vi "add2Parameter.vi"(0 "Enum":T1(ring), 1 "data":variant, 2 "Parameter":variant, 3 "typeDescriptor":string, 5 "error in":errorcluster) -> (16 "Parameter out":variant, 17 "typeDescriptor out":string, 19 "error out":errorcluster)   [LabVIEW 2012, in "HGF_SV.lvlib"]
uses:
  HGF_SV.lvlib
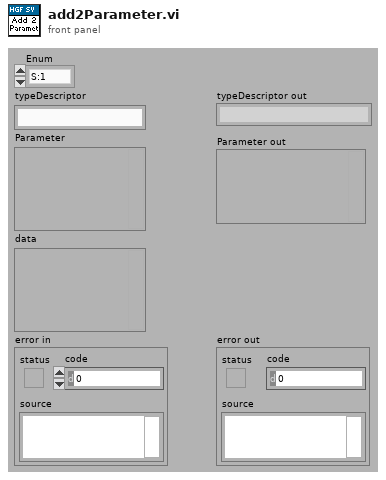
[diagram p1: front panel]
types:
  T1 = enum16{"S:1", "S:2", "L:1", "L:2", "I:1", "I:2", "X:1", "X:2", "F:1", "F:2", "D:1", "D:2", "C"}
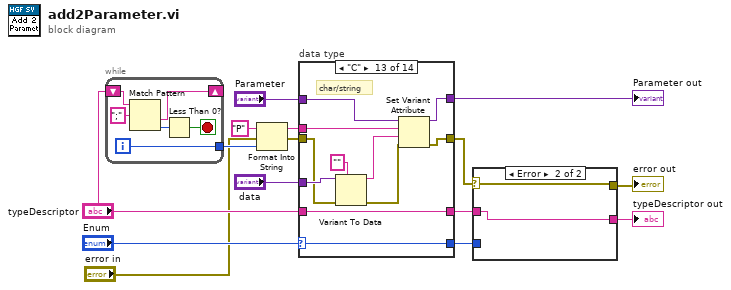
[diagram p0: block diagram]
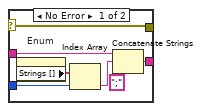
[diagram p2: hidden frame]
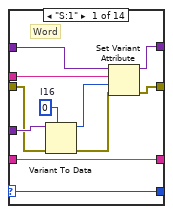
[diagram p3: hidden frame]
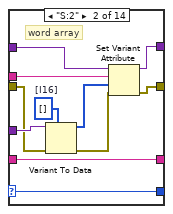
[diagram p4: hidden frame]
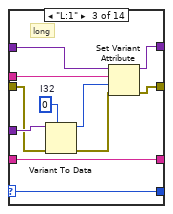
[diagram p5: hidden frame]
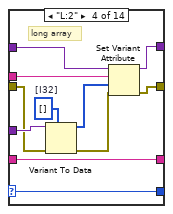
[diagram p6: hidden frame]
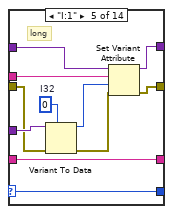
[diagram p7: hidden frame]
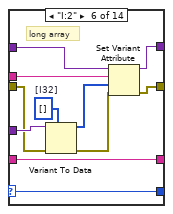
[diagram p8: hidden frame]
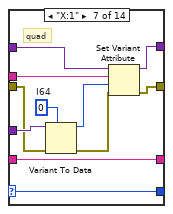
[diagram p9: hidden frame]
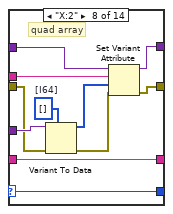
[diagram p10: hidden frame]
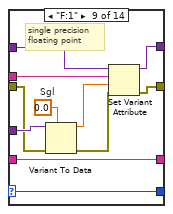
[diagram p11: hidden frame]
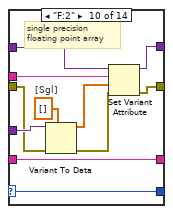
[diagram p12: hidden frame]
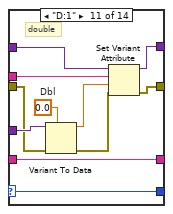
[diagram p13: hidden frame]
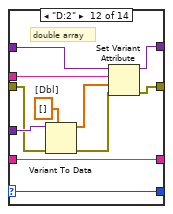
[diagram p14: hidden frame]
diagram:
  n1 = while {
    shift-right: [w19] -> _
    shift-left: "typeDescriptor" -> [w21]
    tunnel: [w16] -> w12
    i -> [w16]
    stop <- w17 stop-if-true
    n2 = Match Pattern(string=w21, regular expression=";") -> (after substring=w19:string, offset past match=w18:i32)  [unwired: 3 out]
    n3 = Less Than 0?(x=w18) -> (x < 0?=w17:bool)
  }
  n4 = Format Into String(initial string="P", error in="error in", w12) -> (resulting string=w10:string, error out=w9:errorcluster)  [unwired: 1 in]
  n5 = case "data type" shown="\"C\"" "Enum" {
    selector: "Enum" -> [w23 w33 w45 w55 w67 w77 w89 w99 w111 w121 w133 w143 w155 w166]
    tunnel: "data" -> [w30 w41 w52 w63 w74 w85 w96 w107 w118 w129 w140 w151 w162 _]
    tunnel: "Parameter" -> [w32 w43 w54 w65 w76 w87 w98 w109 w120 w131 w142 w153 w164 w168]
    tunnel: w10 -> [w31 w42 w53 w64 w75 w86 w97 w108 w119 w130 w141 w152 w163 _]
    tunnel: w9 -> [w28 w38 w50 w60 w72 w82 w94 w104 w116 w126 w138 w148 w160 w165]
    tunnel: [w26 w36 w48 w58 w70 w80 w92 w102 w114 w124 w136 w146 w158 w168] -> w5
    tunnel: [w25 w35 w47 w57 w69 w79 w91 w101 w113 w123 w135 w145 w157 w165] -> w4
    tunnel: "typeDescriptor" -> [w24 w34 w46 w56 w68 w78 w90 w100 w112 w122 w134 w144 w156 w167]
    tunnel: [w24 w34 w46 w56 w68 w78 w90 w100 w112 w122 w134 w144 w156 w167] -> w6
    tunnel: [w23 w33 w45 w55 w67 w77 w89 w99 w111 w121 w133 w143 w155 w166] -> w7
    frame "S:1" {
      w22 = i16 0  # I16
      # "Word"
      n6 = Variant To Data(error in=w28, type=w22, Variant=w30) -> (data=w29:i16, error out=w27:errorcluster)
      n7 = Set Variant Attribute(Variant=w32, name=w31, value=w29, error in=w27) -> (Variant out=w26:variant, error out=w25:errorcluster)  [unwired: 1 out]
    }
    frame "S:2" {
      w40 = i16[] []  # [I16]
      # "word array"
      n8 = Variant To Data(error in=w38, type=w40, Variant=w41) -> (data=w39:i16[], error out=w37:errorcluster)
      n9 = Set Variant Attribute(Variant=w43, name=w42, value=w39, error in=w37) -> (Variant out=w36:variant, error out=w35:errorcluster)  [unwired: 1 out]
    }
    frame "L:1" {
      w44 = 0  # I32
      # "long"
      n10 = Variant To Data(error in=w50, type=w44, Variant=w52) -> (data=w51:i32, error out=w49:errorcluster)
      n11 = Set Variant Attribute(Variant=w54, name=w53, value=w51, error in=w49) -> (Variant out=w48:variant, error out=w47:errorcluster)  [unwired: 1 out]
    }
    frame "L:2" {
      w62 = i32[] []  # [I32]
      # "long array"
      n12 = Variant To Data(error in=w60, type=w62, Variant=w63) -> (data=w61:i32[], error out=w59:errorcluster)
      n13 = Set Variant Attribute(Variant=w65, name=w64, value=w61, error in=w59) -> (Variant out=w58:variant, error out=w57:errorcluster)  [unwired: 1 out]
    }
    frame "I:1" {
      w66 = 0  # I32
      # "long"
      n14 = Variant To Data(error in=w72, type=w66, Variant=w74) -> (data=w73:i32, error out=w71:errorcluster)
      n15 = Set Variant Attribute(Variant=w76, name=w75, value=w73, error in=w71) -> (Variant out=w70:variant, error out=w69:errorcluster)  [unwired: 1 out]
    }
    frame "I:2" {
      w84 = i32[] []  # [I32]
      # "long array"
      n16 = Variant To Data(error in=w82, type=w84, Variant=w85) -> (data=w83:i32[], error out=w81:errorcluster)
      n17 = Set Variant Attribute(Variant=w87, name=w86, value=w83, error in=w81) -> (Variant out=w80:variant, error out=w79:errorcluster)  [unwired: 1 out]
    }
    frame "X:1" {
      w88 = i64 0  # I64
      # "quad"
      n18 = Variant To Data(error in=w94, type=w88, Variant=w96) -> (data=w95:i64, error out=w93:errorcluster)
      n19 = Set Variant Attribute(Variant=w98, name=w97, value=w95, error in=w93) -> (Variant out=w92:variant, error out=w91:errorcluster)  [unwired: 1 out]
    }
    frame "X:2" {
      w106 = i64[] []  # [I64]
      # "quad array"
      n20 = Variant To Data(error in=w104, type=w106, Variant=w107) -> (data=w105:i64[], error out=w103:errorcluster)
      n21 = Set Variant Attribute(Variant=w109, name=w108, value=w105, error in=w103) -> (Variant out=w102:variant, error out=w101:errorcluster)  [unwired: 1 out]
    }
    frame "F:1" {
      w110 = sgl 0.0  # Sgl
      # "single precision \nfloating point"
      n22 = Variant To Data(error in=w116, type=w110, Variant=w118) -> (data=w117:sgl, error out=w115:errorcluster)
      n23 = Set Variant Attribute(Variant=w120, name=w119, value=w117, error in=w115) -> (Variant out=w114:variant, error out=w113:errorcluster)  [unwired: 1 out]
    }
    frame "F:2" {
      w128 = sgl[] []  # [Sgl]
      # "single precision\nfloating point array"
      n24 = Variant To Data(error in=w126, type=w128, Variant=w129) -> (data=w127:sgl[], error out=w125:errorcluster)
      n25 = Set Variant Attribute(Variant=w131, name=w130, value=w127, error in=w125) -> (Variant out=w124:variant, error out=w123:errorcluster)  [unwired: 1 out]
    }
    frame "D:1" {
      w132 = 0.0  # Dbl
      # "double"
      n26 = Variant To Data(error in=w138, type=w132, Variant=w140) -> (data=w139:dbl, error out=w137:errorcluster)
      n27 = Set Variant Attribute(Variant=w142, name=w141, value=w139, error in=w137) -> (Variant out=w136:variant, error out=w135:errorcluster)  [unwired: 1 out]
    }
    frame "D:2" {
      w150 = dbl[] []  # [Dbl]
      # "double array"
      n28 = Variant To Data(error in=w148, type=w150, Variant=w151) -> (data=w149:dbl[], error out=w147:errorcluster)
      n29 = Set Variant Attribute(Variant=w153, name=w152, value=w149, error in=w147) -> (Variant out=w146:variant, error out=w145:errorcluster)  [unwired: 1 out]
    }
    frame "C" {
      # "char/string"
      n30 = Variant To Data(error in=w160, type="", Variant=w162) -> (data=w161:string, error out=w159:errorcluster)
      n31 = Set Variant Attribute(Variant=w164, name=w163, value=w161, error in=w159) -> (Variant out=w158:variant, error out=w157:errorcluster)  [unwired: 1 out]
    }
    frame Default {
    }
  }
  "Parameter out" <- w5
  n32 = case shown="Error" w4 {
    selector: w4 -> [w170 w177]
    tunnel: w7 -> [w174 _]
    tunnel: w6 -> [w173 w176]
    tunnel: [w170 w177] -> w3
    tunnel: [w169 w176] -> w2
    frame No Error {
      n33 = property on="Enum" class="Enum (strict)"() -> ("Strings []"=w175:string[])  [unwired: 2 in, 2 out]
      n34 = Index Array(array=w175, index=w174) -> (element=w172:string)
      n35 = Concatenate Strings(w173, w172, ";" ("string")) -> (w169:string)
    }
    frame Error {
    }
  }
  "error out" <- w3
  "typeDescriptor out" <- w2
